vi "SubVI_Definindo_ROI_esteira.vi"(8 "error in (no error)":errorcluster, 10 "Session in":T2) -> (0 "error out":errorcluster, 1 "ROI Descriptor":T3 {"Contours"."Type" items=["No Selection", "Point", "Line", "Rectangle", "Oval", "Polygon", "Freehand Region", "Annulus", "Unused2", "Unused3", "Broken Line", "Freehand Line", "Rotated Rectangle"]}, 3 "Session Out":T2)   [LabVIEW 2017]
uses:
  <vilib>/userdefined/High Color/IMAQdx.ctl
  <vilib>/vision/Measure.llb/Straight Edge Options.ctl
  <vilib>/vision/Measure.llb/Straight Edge Process.ctl
  <vilib>/vision/Measure.llb/Edge Options.ctl
  <vilib>/vision/Measure.llb/Edge Polarity.ctl
  <vilib>/vision/driver/IMAQdx.llb/IMAQdx Buffer Number Mode.ctl
  <vilib>/vision/NI_Vision_Development_Module.lvlib
  <resource>/objmgr/IMAQImage.rc
  <vilib>/vision/driver/NI_Vision_Acquisition_Software.lvlib
panel:
  out "Imagem Original":T1(plugin-control)
  in  "Blue or Luma or Val or Inten Range":cluster{"Lower value":i32, "Upper value":i32}={"Lower value"=0, "Upper value"=200}
  in  "Green or Sat Range":cluster{"Lower value":i32, "Upper value":i32}={"Lower value"=0, "Upper value"=255}
  in  "Red or Hue Range":cluster{"Lower value":i32, "Upper value":i32}={"Lower value"=0, "Upper value"=255}
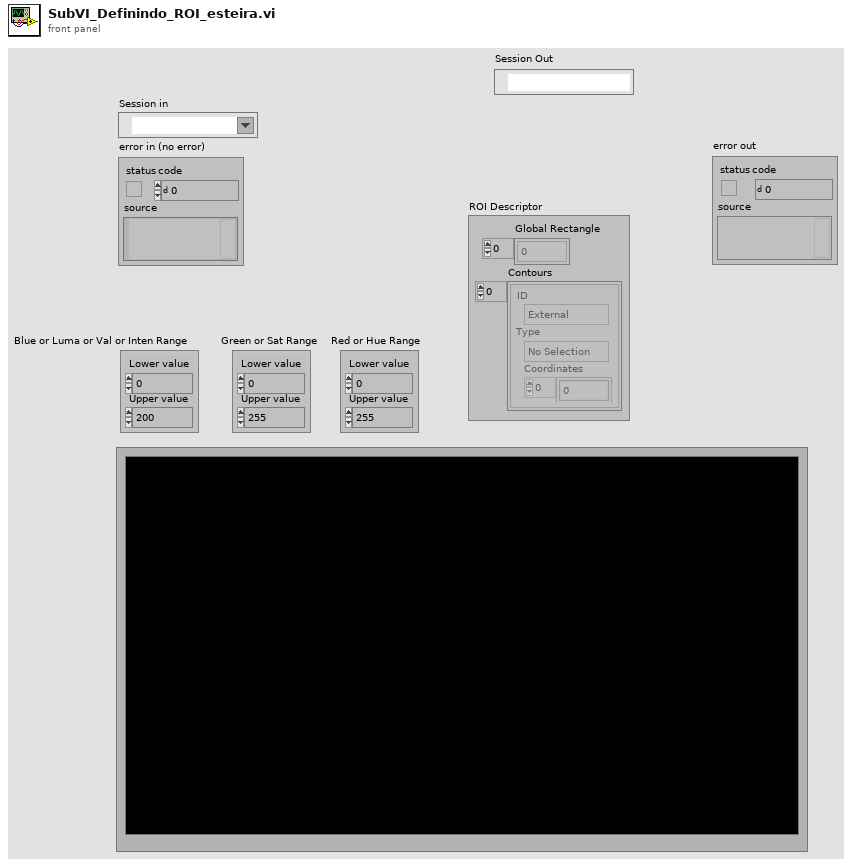
[diagram p1: front panel]
types:
  T1 = typedef "IMAQ Image.ctl" = refnum<image>
  T2 = typedef "IMAQdx.ctl" = refnum<k21>
  T3 = typedef "ROI Descriptor" = cluster{"Global Rectangle":i32[], "Contours":cluster{"ID":enum32{"External", "Internal"}, "Type":u32, "Coordinates":i32[]}[]}
  T4 = typedef "NI_Vision_Acquisition_Software.lvlib/IMAQdx Buffer Number Mode.ctl" = enum32{"Next", "Last", "Buffer Number", "Every", "Last New"}
  T5 = typedef "Edge Options.ctl" = cluster{"Edge Polarity":T6, "Kernel Size":u32, "Width":u32, "Minimum Edge Strength":sgl, "Interpolation Type":enum32{"Zero Order", "Bilinear", "Quadratic", "Cubic", "Bilinear Fixed"}, "Data Processing Method":enum32{"Average", "Median"}}
  T6 = typedef "Edge Polarity.ctl" = u32
  T7 = cluster{"Search Direction":u32, "Edge Options":T5, "Show Search Area":bool, "Show Search Lines":bool, "Show Edges Found":bool, "Show Result":bool, "Search Area Color":u32, "Search Lines Color":u32, "Edge Locations Color":u32, "Result Color":u32, "Overlay Group Name":string}
  T8 = typedef "Straight Edge Options.ctl" = cluster{"Number of Lines":i32, "Type":T9, "Min. Score":dbl, "Max. Score":dbl, "Orientation":dbl, "Angle Range":dbl, "Angle Tolerance":dbl, "Step Size":u32, "Min. SNR (db)":dbl, "Min. Points (%)":dbl, "Hough Iterations":i32}
  T9 = typedef "Straight Edge Process.ctl" = enum32{"First Edge Rake", "Best Edge Rake", "Hough Edge Rake", "First Edge Projection", "Best Edge Projection"}
  T10 = cluster{"element":dbl, "y":i32, "x":i32, "element":dbl, "element":dbl}
  T11 = cluster{"Point1 (Pixels)":cluster{"X":sgl, "Y":sgl}, "Point2 (Pixels)":cluster{"X":sgl, "Y":sgl}, "Point1 (Real-World)":cluster{"X":sgl, "Y":sgl}, "Point2 (Real-World)":cluster{"X":sgl, "Y":sgl}, "Angle (Pixel)":dbl, "Angle (Real-World)":dbl, "Score":dbl, "Straightness":dbl, "Average SNR (db)":dbl, "Calibration Valid":bool}[]
  T12 = cluster{"Point1 (Pixels)":cluster{"X":sgl, "Y":sgl}, "Point2 (Pixels)":cluster{"X":sgl, "Y":sgl}, "Point1 (Real-World)":cluster{"X":sgl, "Y":sgl}, "Point2 (Real-World)":cluster{"X":sgl, "Y":sgl}, "Angle (Pixel)":dbl, "Angle (Real-World)":dbl, "Score":dbl, "Straightness":dbl, "Average SNR (db)":dbl, "Calibration Valid":bool}
  T13 = cluster{"element":dbl, sgl, "x":i32, sgl, "element":dbl}
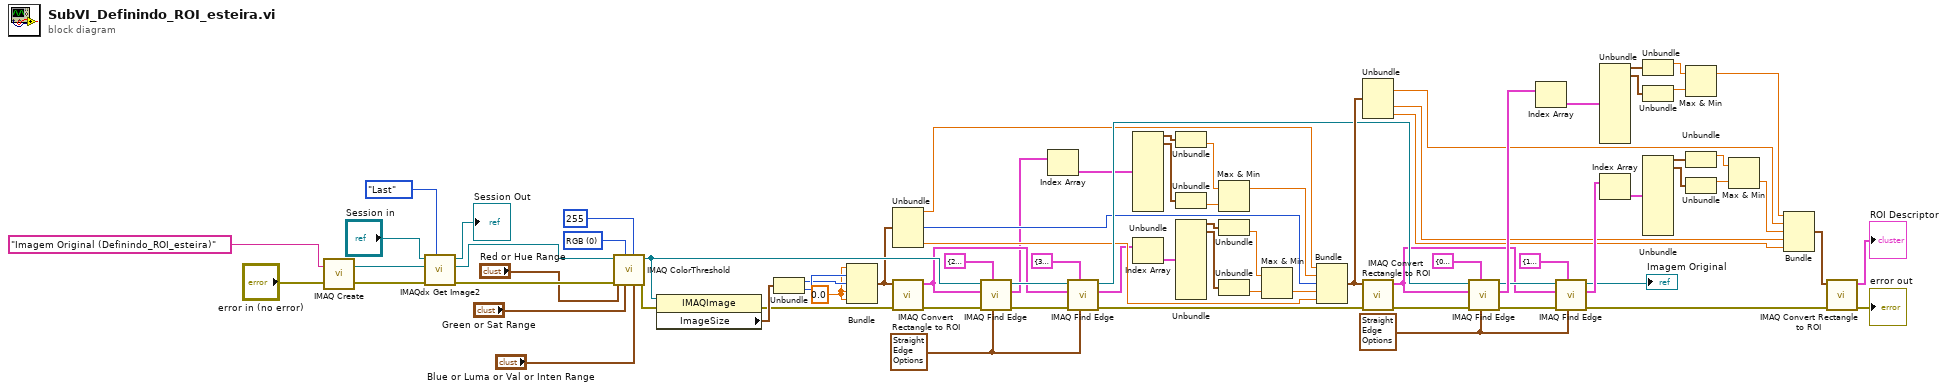
[diagram p0: block diagram]
diagram:
  w23 = u16 0 items=["RGB", "HSL", "HSV", "HSI"] ("Color Mode")
  w56 = T8 {"Number of Lines"=1, "Type"=enum."First Edge Rake", "Min. Score"=10.0, "Max. Score"=1000.0, "Orientation"=0.0, "Angle Range"=45.0, "Angle Tolerance"=1.0, "Step Size"=32, "Min. SNR (db)"=0.0, "Min. Points (%)"=25.0, "Hough Iterations"=5} ("Fit Options")
  w31 = T8 {"Number of Lines"=1, "Type"=enum."First Edge Rake", "Min. Score"=10.0, "Max. Score"=1000.0, "Orientation"=0.0, "Angle Range"=45.0, "Angle Tolerance"=1.0, "Step Size"=32, "Min. SNR (db)"=0.0, "Min. Points (%)"=25.0, "Hough Iterations"=5} ("Fit Options")
  w26 = 0.0 ("element")
  n1 = call "IMAQ Create"("Image Name"="Imagem Original (Definindo_ROI_esteira)", "error in (no error)"="error in (no error)") -> ("New Image"=w20:T1, "error out"=w7:errorcluster)  [unwired: 3 in]
  n2 = call <vilib>:"IMAQdx Get Image2.vi"("Buffer Number Mode (Next)"=IMAQdx_Buffer_Number_Mode."Last", "error in"=w7, "Image In"=w20, "Session In"="Session in") -> ("error out"=w17:errorcluster, "Image Out"=w8:T1, "Session Out"=→"Session Out":T2)  [unwired: 4 in, 1 out]
  n3 = call "IMAQ ColorThreshold"("Blue or Luma or Val or Inten Range"="Blue or Luma or Val or Inten Range", "Replace Value"=255, "Green or Sat Range"="Green or Sat Range", "Color Mode"=w23, "error in (no error)"=w17, "Red or Hue Range"="Red or Hue Range", "Image Src"=w8) -> ("error out"=w2:errorcluster, "Image Dst Out"=w78:T1)  [unwired: 1 in, 2 out]
  n4 = property class="IMAQImage"(reference=w78, error in=w2) -> (error out=w16:errorcluster, "ImageSize"=w25:cluster{"x":i32, "y":i32})  [unwired: 1 out]
  n5 = Unbundle(w25) -> ("x"=w28:i32, "y"=w29:i32)
  n6 = Bundle("element"=w26, "y"=w29, "x"=w28, "element"=w26, "element"=w26) -> (w58:T10)  [unwired: 1 in]
  n7 = Unbundle(w58) -> ("element"=w49:dbl, "x"=w48:i32, "element"=w50:dbl)  [unwired: 2 out]
  n8 = call "IMAQ Convert Rectangle to ROI"("error in (no error)"=w16, "Rectangle"=w58) -> ("error out"=w15:errorcluster, "ROI Descriptor"=w32:T3)  [unwired: 7 in]
  n9 = call "IMAQ Find Edge"("Line Fit Options"=w31, "Options"=T7 {"Search Direction"=2, "Edge Options"={"Edge Polarity"=2, "Kernel Size"=3, "Width"=1, "Minimum Edge Strength"=80.0, "Interpolation Type"=enum."Bilinear Fixed", "Data Processing Method"=enum."Average"}, "Show Search Area"=FALSE, "Show Search Lines"=FALSE, "Show Edges Found"=FALSE, "Show Result"=TRUE, "Search Area Color"=65280, "Search Lines Color"=255, "Edge Locations Color"=16776960, "Result Color"=16711680, "Overlay Group Name"=""}, "error in (no error)"=w15, "ROI Descriptor"=w32, "Image"=w78) -> ("error out"=w14:errorcluster, "Straight Edges"=w30:T11, "Image Out"=w33:T1)  [unwired: 1 in, 3 out]
  n10 = Index Array(array=w30) -> (element=w36:T12)  [unwired: 1 in]
  n11 = call "IMAQ Find Edge"("Line Fit Options"=w31, "Options"=T7 {"Search Direction"=3, "Edge Options"={"Edge Polarity"=2, "Kernel Size"=3, "Width"=1, "Minimum Edge Strength"=80.0, "Interpolation Type"=enum."Bilinear Fixed", "Data Processing Method"=enum."Average"}, "Show Search Area"=FALSE, "Show Search Lines"=FALSE, "Show Edges Found"=FALSE, "Show Result"=TRUE, "Search Area Color"=65280, "Search Lines Color"=255, "Edge Locations Color"=16776960, "Result Color"=16711680, "Overlay Group Name"=""}, "error in (no error)"=w14, "ROI Descriptor"=w32, "Image"=w33) -> ("error out"=w13:errorcluster, "Straight Edges"=w35:T11, "Image Out"=w55:T1)  [unwired: 1 in, 3 out]
  n12 = Unbundle(w36) -> ("Point1 (Pixels)"=w38:cluster{"X":sgl, "Y":sgl}, "Point2 (Pixels)"=w39:cluster{"X":sgl, "Y":sgl})  [unwired: 8 out]
  n13 = Index Array(array=w35) -> (element=w37:T12)  [unwired: 1 in]
  n14 = Unbundle(w38) -> ("Y"=w42:sgl)  [unwired: 1 out]
  n15 = Unbundle(w39) -> ("Y"=w43:sgl)  [unwired: 1 out]
  n16 = Unbundle(w37) -> ("Point1 (Pixels)"=w40:cluster{"X":sgl, "Y":sgl}, "Point2 (Pixels)"=w41:cluster{"X":sgl, "Y":sgl})  [unwired: 8 out]
  n17 = Max & Min(x=w42, y=w43) -> (max(x,y)=w46:sgl)  [unwired: 1 out]
  n18 = Unbundle(w40) -> ("Y"=w44:sgl)  [unwired: 1 out]
  n19 = Unbundle(w41) -> ("Y"=w45:sgl)  [unwired: 1 out]
  n20 = Max & Min(x=w44, y=w45) -> (min(x,y)=w47:sgl)  [unwired: 1 out]
  n21 = Bundle("element"=w49, w46, "x"=w48, w47, "element"=w50) -> (w60:T13)  [unwired: 1 in]
  n22 = Unbundle(w60) -> (w61:sgl, w62:sgl, "element"=w59:dbl)  [unwired: 2 out]
  n23 = call "IMAQ Convert Rectangle to ROI"("error in (no error)"=w13, "Rectangle"=w60) -> ("error out"=w12:errorcluster, "ROI Descriptor"=w53:T3)  [unwired: 7 in]
  n24 = call "IMAQ Find Edge"("Line Fit Options"=w56, "Options"=T7 {"Search Direction"=0, "Edge Options"={"Edge Polarity"=2, "Kernel Size"=3, "Width"=1, "Minimum Edge Strength"=80.0, "Interpolation Type"=enum."Bilinear Fixed", "Data Processing Method"=enum."Average"}, "Show Search Area"=FALSE, "Show Search Lines"=FALSE, "Show Edges Found"=FALSE, "Show Result"=TRUE, "Search Area Color"=65280, "Search Lines Color"=255, "Edge Locations Color"=16776960, "Result Color"=16711680, "Overlay Group Name"=""}, "error in (no error)"=w12, "ROI Descriptor"=w53, "Image"=w55) -> ("error out"=w11:errorcluster, "Straight Edges"=w69:T11, "Image Out"=w54:T1)  [unwired: 1 in, 3 out]
  n25 = Index Array(array=w69) -> (element=w65:T12)  [unwired: 1 in]
  n26 = call "IMAQ Find Edge"("Line Fit Options"=w56, "Options"=T7 {"Search Direction"=1, "Edge Options"={"Edge Polarity"=2, "Kernel Size"=3, "Width"=1, "Minimum Edge Strength"=80.0, "Interpolation Type"=enum."Bilinear Fixed", "Data Processing Method"=enum."Average"}, "Show Search Area"=FALSE, "Show Search Lines"=FALSE, "Show Edges Found"=FALSE, "Show Result"=TRUE, "Search Area Color"=65280, "Search Lines Color"=255, "Edge Locations Color"=16776960, "Result Color"=16711680, "Overlay Group Name"=""}, "error in (no error)"=w11, "ROI Descriptor"=w53, "Image"=w54) -> ("error out"=w10:errorcluster, "Straight Edges"=w70:T11, "Image Out"=→"Imagem Original":T1)  [unwired: 1 in, 3 out]
  n27 = Unbundle(w65) -> ("Point1 (Pixels)"=w64:cluster{"X":sgl, "Y":sgl}, "Point2 (Pixels)"=w63:cluster{"X":sgl, "Y":sgl})  [unwired: 8 out]
  n28 = Index Array(array=w70) -> (element=w66:T12)  [unwired: 1 in]
  n29 = Unbundle(w64) -> ("X"=w73:sgl)  [unwired: 1 out]
  n30 = Unbundle(w63) -> ("X"=w74:sgl)  [unwired: 1 out]
  n31 = Unbundle(w66) -> ("Point1 (Pixels)"=w67:cluster{"X":sgl, "Y":sgl}, "Point2 (Pixels)"=w68:cluster{"X":sgl, "Y":sgl})  [unwired: 8 out]
  n32 = Max & Min(x=w73, y=w74) -> (max(x,y)=w71:sgl)  [unwired: 1 out]
  n33 = Unbundle(w67) -> ("X"=w75:sgl)  [unwired: 1 out]
  n34 = Unbundle(w68) -> ("X"=w76:sgl)  [unwired: 1 out]
  n35 = Max & Min(x=w75, y=w76) -> (min(x,y)=w72:sgl)  [unwired: 1 out]
  n36 = Bundle(w71, w61, w72, w62, "element"=w59) -> (w57:cluster{sgl, sgl, sgl, sgl, "element":dbl})  [unwired: 1 in]
  n37 = call "IMAQ Convert Rectangle to ROI"("error in (no error)"=w10, "Rectangle"=w57) -> ("error out"=→"error out":errorcluster, "ROI Descriptor"=→"ROI Descriptor":T3)  [unwired: 7 in]
